vi "Drive Used GB.vi"(8 "error in (no error)":errorcluster, 10 "Path":path, 11 "Windows System SAL in":refnum<class "Windows System SAL.lvclass">) -> (0 "error out":errorcluster, 2 "Used GB":dbl, 3 "Windows System SAL out":refnum<class "Windows System SAL.lvclass">)   [LabVIEW 2020, in "Volatus.lvlib" / "Windows System SAL.lvclass"]
uses:
  Windows System SAL.lvclass
  Windows System SAL.lvclass/Windows System SAL.ctl
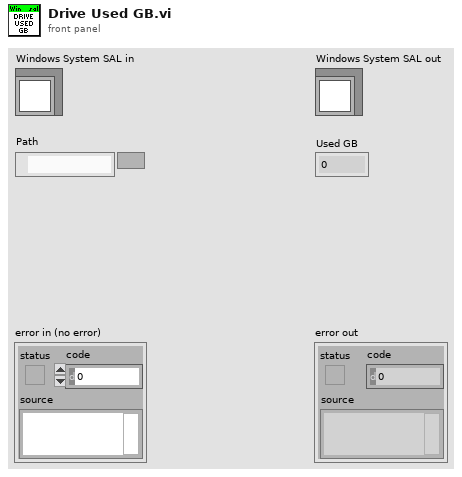
[diagram p1: front panel]
types:
  T1 = typedef "Volatus.lvlib/Windows System SAL.lvclass/Drive Info.ctl" = cluster{"Size GB":dbl, "Free GB":dbl}
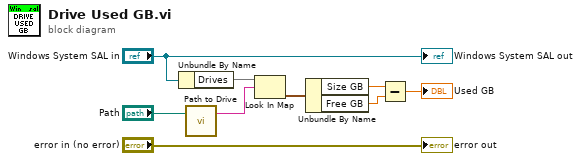
[diagram p0: block diagram]
diagram:
  n1 = Unbundle By Name("Windows System SAL in") -> ("Drives"=w8:map{string, T1})
  n2 = call "Path to Drive.vi"("Path"="Path") -> ("Drive"=w7:string)  [unwired: 6 in]
  n3 = Look In Map(map=w8, key=w7) -> (value=w6:T1)  [unwired: 1 in, 1 out]
  n4 = Unbundle By Name(w6) -> ("Size GB"=w3:dbl, "Free GB"=w2:dbl)
  n5 = Subtract(x=w3, y=w2) -> (x-y=→"Used GB":dbl)
  "error out" <- "error in (no error)"
  "Windows System SAL out" <- "Windows System SAL in"
